vi "Day10-1.vi"() -> ()   [LabVIEW 2021]
panel:
  out "sum":u64
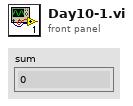
[diagram p1: front panel]
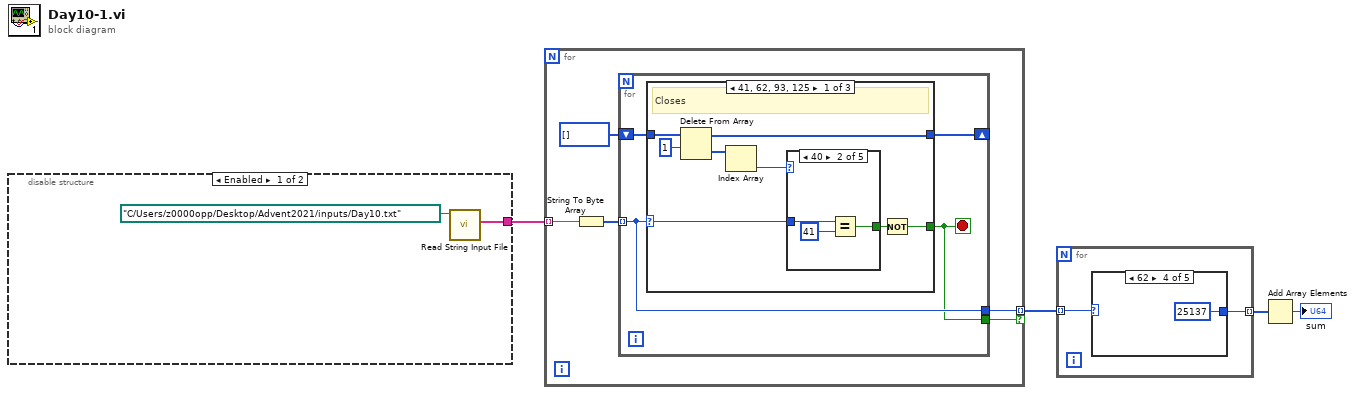
[diagram p0: block diagram]
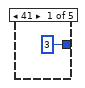
[diagram p2: hidden frame]
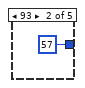
[diagram p3: hidden frame]
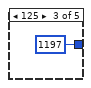
[diagram p4: hidden frame]
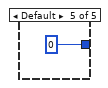
[diagram p5: hidden frame]
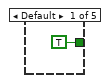
[diagram p6: hidden frame]
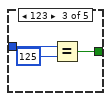
[diagram p7: hidden frame]
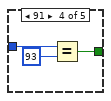
[diagram p8: hidden frame]
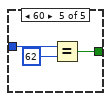
[diagram p9: hidden frame]
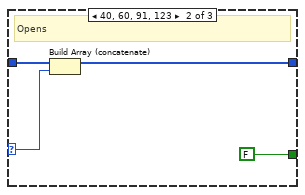
[diagram p10: hidden frame]
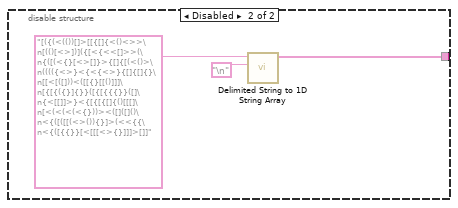
[diagram p12: hidden frame]
diagram:
  n1 = disable-structure shown="Enabled" {
    disable-tunnel: [w5 w7] -> w4
    frame Enabled {
      n2 = call "Read String Input File.vi"("file path (dialog if empty)"=path "C:/Users/z0000opp/Desktop/Advent2021/inputs/Day10.txt") -> ("input values"=w5:string[])  [unwired: 10 in]
    }
    frame Disabled {
      n3 = call <vilib>:"Delimited String to 1D String Array.vi"("delimiter"="\n", "delimited string"="[({(<(())[]>[[{[]{<()<>>\n[(()[<>])]({[<{<<[]>>(\n{([(<{}[<>[]}>{[]{[(<()>\n(((({<>}<{<{<>}{[]{[]{}\n[[<[([]))<([[{}[[()]]]\n[{[{({}]{}}([{[{{{}}([]\n{<[[]]>}<{[{[{[]{()[[[]\n[<(<(<(<{}))><([]([]()\n<{([([[(<>()){}]>(<<{{\n<{([{{}}[<[[[<>{}]]]>[]]") -> ("string array"=w7:string[])  [unwired: 9 in]
    }
  }
  n4 = for {
    tunnel: w4 -> [w14] mode=indexing
    tunnel: [w11] -> w3 mode=indexing if=w10
    n5 = String To Byte Array(string=w14) -> (unsigned byte array=w13:u8[])
    n6 = for {
      tunnel: w13 -> [w16] mode=indexing
      shift-right: [w17] -> _
      shift-left: u8[] [] -> [w18]
      tunnel: [w16] -> w11
      tunnel: [w15] -> w10
      stop <- w15 stop-if-true
      n7 = case shown="41, 62, 93, 125" w16 {
        selector: w16 -> [w21 w42 _]
        tunnel: w18 -> [w26 w43 w44]
        tunnel: [w24 w41 w44] -> w17
        tunnel: [w19 FALSE _] -> w15
        frame 41, 62, 93, 125 {
          # "Closes"
          n8 = Delete From Array(array=w26, length=1) -> (deleted portion=w23:u8[], array with subset deleted=w24:u8[])  [unwired: 1 in]
          n9 = Index Array(array=w23) -> (element=w22:u8)  [unwired: 1 in]
          n10 = case shown="40" w22 {
            tunnel: w21 -> [_ w30 w33 w36 w39]
            tunnel: [TRUE w28 w31 w34 w37] -> w20
            frame Default {
            }
            frame 40 {
              n11 = Equal?(x=w30, y=u8 41) -> (x = y?=w28:bool)
            }
            frame 123 {
              n12 = Equal?(x=w33, y=u8 125) -> (x = y?=w31:bool)
            }
            frame 91 {
              n13 = Equal?(x=w36, y=u8 93) -> (x = y?=w34:bool)
            }
            frame 60 {
              n14 = Equal?(x=w39, y=u8 62) -> (x = y?=w37:bool)
            }
          }
          n15 = Not(x=w20) -> (.not. x?=w19:bool)
        }
        frame 40, 60, 91, 123 {
          # "Opens"
          n16 = Build Array (concatenate)(w43, w42) -> (w41:u8[])
        }
        frame Default {
        }
      }
    }
  }
  n17 = for {
    tunnel: w3 -> [w46] mode=indexing
    tunnel: [w45] -> w2 mode=indexing
    n18 = case shown="62" w46 {
      tunnel: [u64 3 u64 57 u64 1197 u64 25137 u64 0] -> w45
      frame 41 {
      }
      frame 93 {
      }
      frame 125 {
      }
      frame 62 {
      }
      frame Default {
      }
    }
  }
  n19 = Add Array Elements(numeric array=w2) -> (sum=→"sum":u64)
